vi "Linear.vi"(0 "controller in":refnum<k24>, 5 "axis names":string[](array[string]), 7 "distances":dbl[](array[numeric]), 9 "speed":dbl, 11 "error in (no error)":errorcluster, 12 "return immediately":bool) -> (4 "controller out":refnum<k24>, 15 "error out":errorcluster)   [LabVIEW 2010]
uses:
  c:/aerotech/controller/5.xx.xxx/ensemble/pc/labview/2010/bin/Aerotech.Ensemble.dll
  bin/Aerotech.Ensemble.dll
  c:/aerotech/controller/5.xx.xxx/ensemble/pc/labview/2010/bin/Aerotech.Ensemble.LabVIEW.dll
  bin/Aerotech.Ensemble.LabVIEW.dll
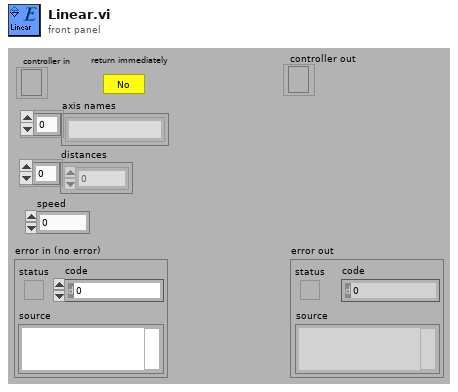
[diagram p1: front panel]
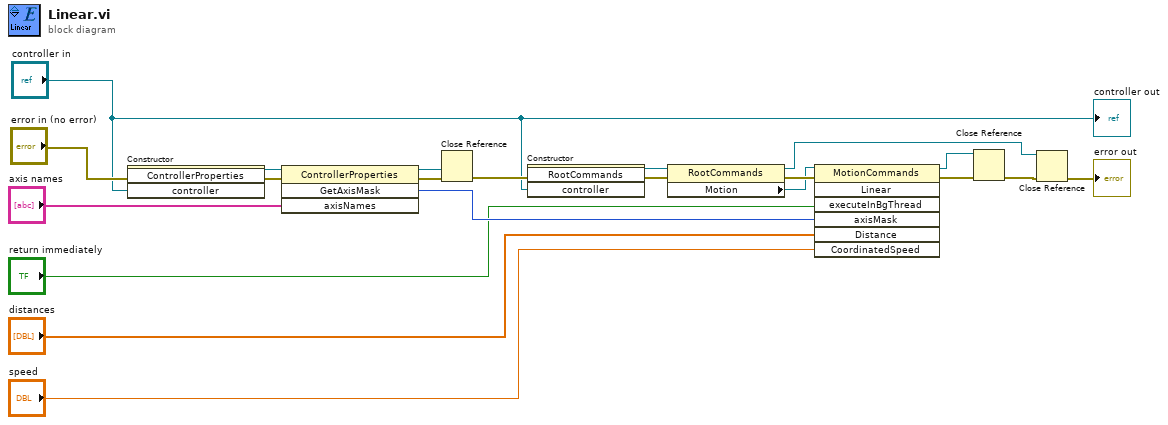
[diagram p0: block diagram]
diagram:
  n1 = constructor class="ControllerProperties"(error in="error in (no error)", "controller"="controller in") -> (reference out=w20:refnum<k24>, error out=w19:errorcluster)  [unwired: 2 in, 2 out]
  n2 = invoke class="ControllerProperties" method="GetAxisMask"(reference=w20, error in=w19, "axisNames"="axis names") -> (reference out=w17:refnum<k24>, error out=w18:errorcluster, "GetAxisMask"=w16:i32)  [unwired: 1 in, 1 out]
  n3 = Close Reference(reference=w17, error in (no error)=w18) -> (error out=w11:errorcluster)
  n4 = constructor class="RootCommands"(error in=w11, "controller"="controller in") -> (reference out=w5:refnum<k24>, error out=w6:errorcluster)  [unwired: 2 in, 2 out]
  n5 = property class="RootCommands"(reference=w5, error in=w6) -> (reference out=w2:refnum<k24>, error out=w4:errorcluster, "Motion"=w3:refnum<k24>)
  n6 = invoke class="MotionCommands" method="Linear"(reference=w3, error in=w4, "executeInBgThread"="return immediately", "axisMask"=w16, "Distance"="distances", "CoordinatedSpeed"="speed") -> (reference out=w8:refnum<k24>, error out=w7:errorcluster)  [unwired: 1 in, 5 out]
  n7 = Close Reference(reference=w8, error in (no error)=w7) -> (error out=w9:errorcluster)
  n8 = Close Reference(reference=w2, error in (no error)=w9) -> (error out=→"error out":errorcluster)
  "controller out" <- "controller in"
